vi "20170502127惠雨6.vi"() -> ()   [LabVIEW 2017]
panel:
  out "波形图":dbl[](graph)
  out "URL":string
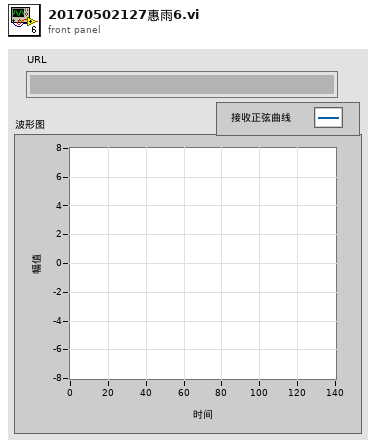
[diagram p1: front panel]
types:
  T1 = cluster{"Sinusoidal Pattern":dbl[], dbl, "停止":bool}
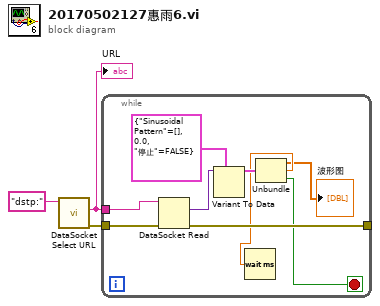
[diagram p0: block diagram]
diagram:
  n1 = call <vilib>:"DataSocket Select URL.vi"("StartURL (empty)"="dstp:") -> ("error out"=w2:errorcluster, "URL"=w3:string)  [unwired: 8 in, 1 out]
  "URL" <- w3
  n2 = while {
    tunnel: w3 -> [w12]
    tunnel: w2 -> [w11]
    tunnel: [w9] -> _
    stop <- w6 stop-if-true
    n3 = DataSocket Read(8:w11, 11:w12) -> (0:w9:errorcluster, 2:w10:variant)  [unwired: 3 in, 5 out]
    n4 = Variant To Data ("变体至数据转换")(type=T1 {"Sinusoidal Pattern"=[], 0.0, "停止"=FALSE} ("输出簇"), Variant=w10) -> (data=w7:T1)  [unwired: 1 in, 1 out]
    n5 = Unbundle(w7) -> ("Sinusoidal Pattern"=→"波形图":dbl[], w5:dbl, "停止"=w6:bool)
    n6 = Wait (ms)(milliseconds to wait=w5) -> ()  [unwired: 1 out]
  }
